vi "Method.vi"(4 "Value":refnum<class "Abs_Double Float.lvclass">) -> (1 "Result":refnum<class "Abs_Boolean.lvclass">)   [LabVIEW 2021, in "Less 0_DBL.lvclass"]
uses:
  Less 0_DBL.lvclass
  Abs_Types/Double Float/Abs_Double Float.lvclass
  Abs_Types/Boolean/Abs_Boolean.lvclass
  C:/TSA/LV_Abstract/Source/Functions/Support/Compare/One Term/DBL/AbsComp_One Term_DBL.lvclass
  C:/Program Files (x86)/National Instruments/LabVIEW 2021/vi.lib/TSA/Abstract Data Classes/Abs_Types/Boolean/Abs_Boolean.lvclass
  Support/Compare/One Term/DBL/AbsComp_One Term_DBL.lvclass/AbsComp_One Term_DBL.ctl
  Support/Compare/One Term/DBL/Properties/Write Numeric A.vi
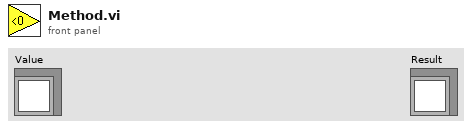
[diagram p1: front panel]
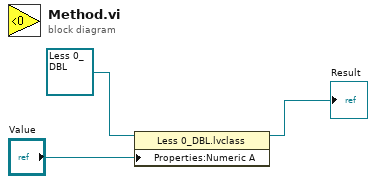
[diagram p0: block diagram]
diagram:
  n1 = property class="Less 0_DBL.lvclass"(reference=refnum<class "Less 0_DBL.lvclass"> refnum ("Greater 0_U64.lvclass"), "Properties:Numeric A"="Value") -> (reference out=→"Result":refnum<class "Less 0_DBL.lvclass">)  [unwired: 1 in, 1 out]
